vi "Set Default Printer.vi"(8 "error in (no error)":errorcluster, 11 "Printer Name":string) -> (0 "error out":errorcluster)   [LabVIEW 2017]
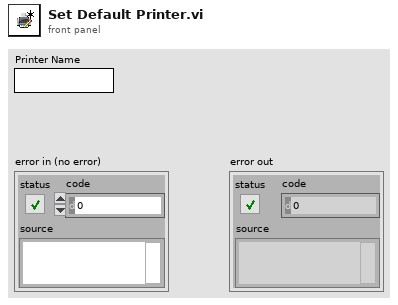
[diagram p1: front panel]
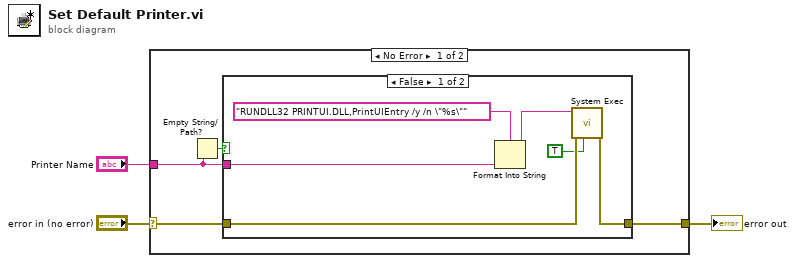
[diagram p0: block diagram]
diagram:
  n1 = case shown="No Error" "error in (no error)" {
    selector: "error in (no error)" -> [w7 w15]
    tunnel: [w6 w15] -> w2
    tunnel: "Printer Name" -> [w4 _]
    frame No Error {
      n2 = Empty String/Path?(string/path=w4) -> (empty?=w5:bool)
      n3 = case shown="False" w5 {
        tunnel: w7 -> [w13 w14]
        tunnel: [w12 w14] -> w6
        tunnel: w4 -> [w9 _]
        frame False {
          n4 = Format Into String(format string="RUNDLL32 PRINTUI.DLL,PrintUIEntry /y /n \"%s\"" ("command line"), w9) -> (resulting string=w8:string)  [unwired: 2 in, 1 out]
          n5 = call <vilib>:"System Exec.vi"("run minimized? (F)"=TRUE, "error in (no error)"=w13, "command line"=w8) -> ("error out"=w12:errorcluster)  [unwired: 5 in, 3 out]
        }
        frame True {
        }
      }
    }
    frame Error {
    }
  }
  "error out" <- w2
